vi "Polling Logging Data From PLC.vi"(7 "Polling Data Input":T1, 8 "error in (no error)":errorcluster, 11 "TCP Network Connection in":refnum<k5>) -> (0 "error out":errorcluster, 1 "Data Read":u8[][](array[numeric]), 2 "PLC Data out":T1, 3 "TCP Network Connection out":refnum<k5>, 4 "Elapsed Time(ms)":u32, 5 "Float Data Valid?":bool[](array[boolean]), 6 "Motor2RatingRPM":u16)   [LabVIEW 2018]
uses:
  Ctls/DisplayIndicator.ctl
  Ctls/MotroConfigData.ctl
  Ctls/MotorConfig.ctl
  Ctls/MagType.ctl
  Siemens S7 TCP v3_3 LV 8_5/Siemens S7 TCP v3_3 LV 8_5/S7 TCP API Library/S7 TCP.lvlib
panel:
  out "Motor1RatingRPM":u16
  out "Bool Data Valid":bool
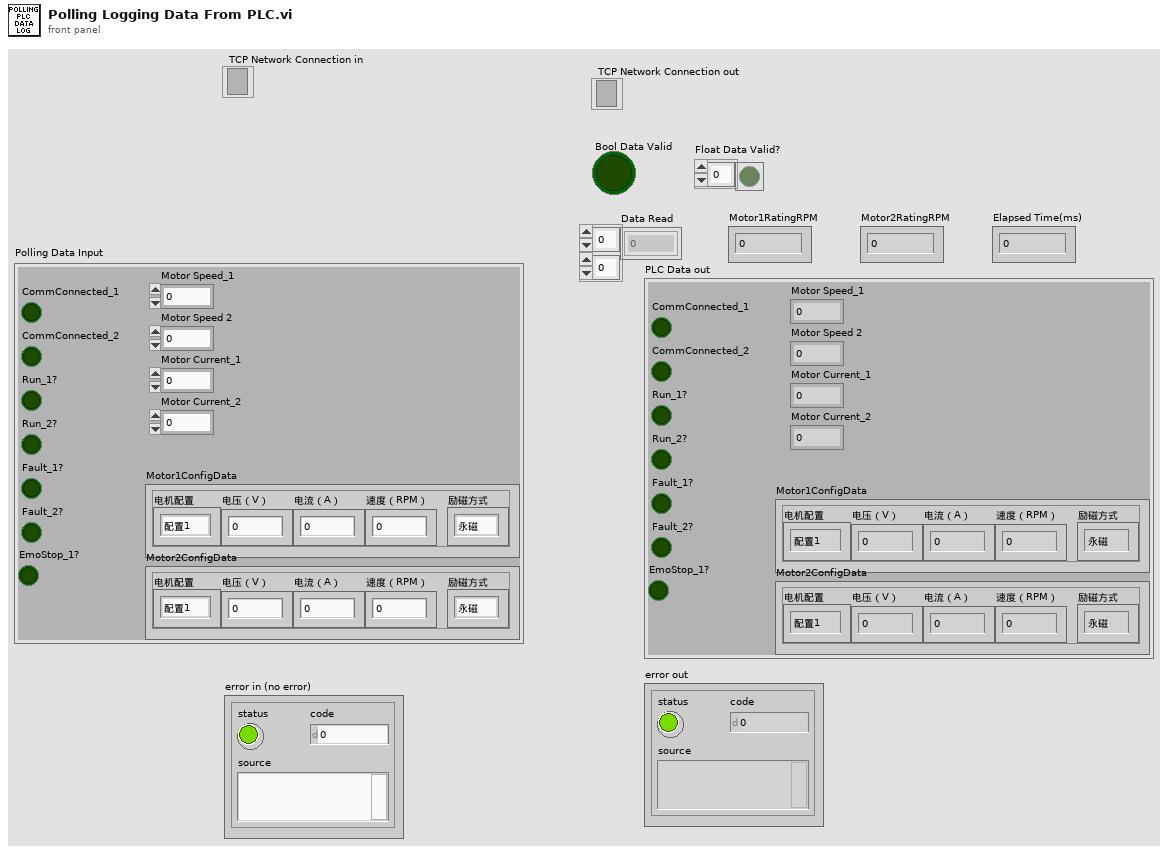
[diagram p1: front panel]
types:
  T1 = typedef "DisplayIndicator.ctl" = cluster{"CommConnected_1":bool, "Run_1?":bool, "Fault_1?":bool, "CommConnected_2":bool, "Run_2?":bool, "Fault_2?":bool, "Motor Speed 2":sgl, "Motor Speed_1":sgl, "Motor Current_1":sgl, "Motor Current_2":sgl, "Motor1ConfigData":T2, "Motor2ConfigData":T2, "EmoStop_1?":bool}
  T2 = typedef "MotroConfigData.ctl" = cluster{"电机配置":T3, "电压（V）":dbl, "电流（A）":dbl, "速度（RPM）":dbl, "励磁方式":T4}
  T3 = typedef "MotorConfig.ctl" = enum16{"配置1", "配置2", "配置3", "配置4"}
  T4 = typedef "MagType.ctl" = enum16{"永磁", "励磁"}
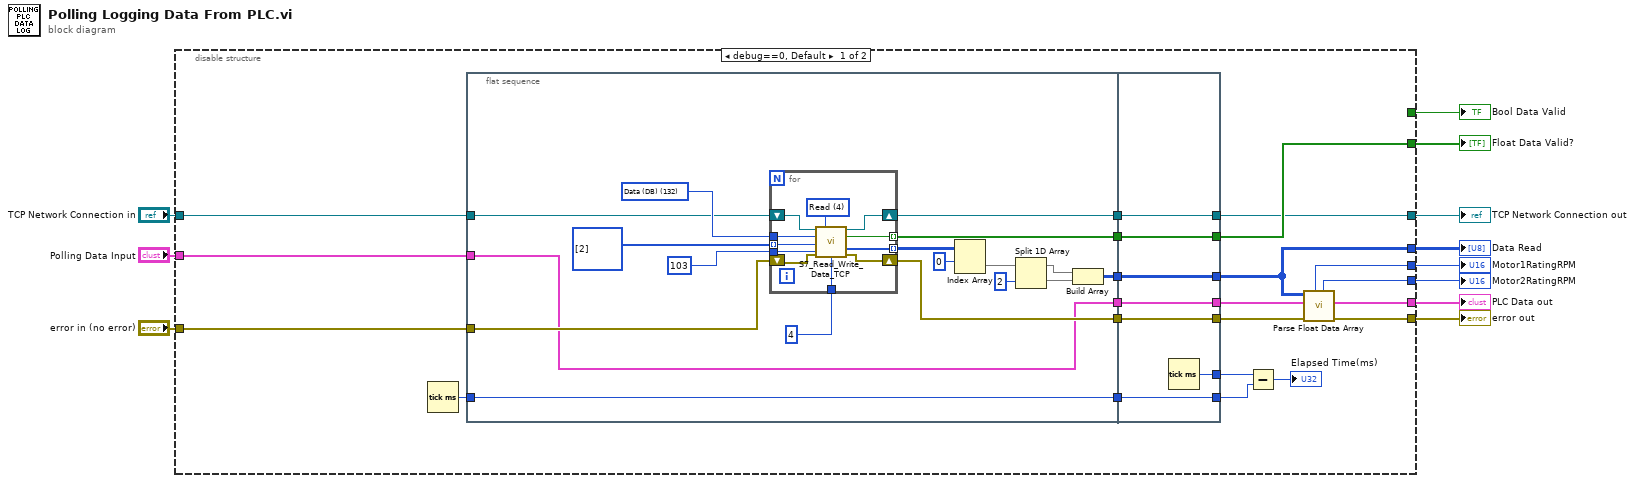
[diagram p0: block diagram]
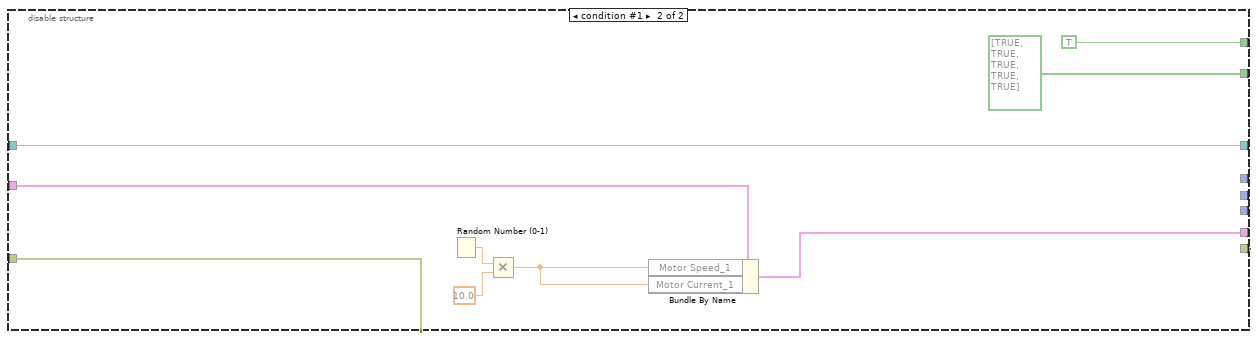
[diagram p2: hidden frame]
diagram:
  n1 = disable-structure shown="debug==0, Default" {
    disable-tunnel: [w33 w75] -> w11
    disable-tunnel: [w32 w71] -> w10
    disable-tunnel: [w24 _] -> w9
    disable-tunnel: [w31 bool[] [TRUE, TRUE, TRUE, TRUE, TRUE]] -> w8
    disable-tunnel: [w30 w78] -> w7
    disable-tunnel: [_ TRUE ("Data Valid")] -> w6
    disable-tunnel: "TCP Network Connection in" -> [w27 w78]
    disable-tunnel: "error in (no error)" -> [w25 w71]
    disable-tunnel: [w29 _] -> w3
    disable-tunnel: [w28 _] -> w2
    disable-tunnel: "Polling Data Input" -> [w23 w70]
    frame condition #0 (active) {
      n2 = Tick Count (ms)() -> (millisecond timer value=w16:u32)
      n3 = flat-sequence {
        tunnel: w27 -> [w45]
        tunnel: w25 -> [w43]
        tunnel: w23 -> [w35]
        tunnel: [w51] -> w21
        tunnel: [w48] -> w20
        tunnel: [w44] -> w19
        tunnel: [w36] -> w18
        tunnel: [w35] -> w17
        tunnel: w16 -> [w34]
        tunnel: [w34] -> w15
        tunnel: [w65] -> w22
        tunnel: [w66] -> w24
        tunnel: [w67] -> w26
        tunnel: [w68] -> w30
        tunnel: [w69] -> w31
        tunnel: w21 -> [w69]
        tunnel: w20 -> [w68]
        tunnel: w19 -> [w67]
        tunnel: w18 -> [w66]
        tunnel: w17 -> [w65]
        tunnel: [w64] -> w14
        tunnel: w15 -> [w63]
        tunnel: [w63] -> w13
        frame #0 {
          w47 = u8 132 items=["I/O (P)"=128, "Input (I)"=129, "Output (Q)"=130, "Bit Memory (M)"=131, "Data (DB)"=132, "Instance Data (DI)"=133, "Local Data (L)"=134, "Predecessor Local Data (VL)"=135] ("Address Areas")
          n4 = for {
            tunnel: w47 -> [w61]
            tunnel: u16 103 ("Data Block #") -> [w58]
            tunnel: u32[] [2] -> [w57] mode=indexing
            tunnel: u16 4 ("Length (bytes)") -> [w56]
            tunnel: [w55] -> w51 mode=indexing
            tunnel: [w54] -> w42 mode=indexing
            shift-right: [w52] -> w44
            shift-left: w43 -> [w53]
            shift-right: [w59] -> w48
            shift-left: w45 -> [w62]
            w60 = u8 4 items=["Read"=4, "Write"=5] ("Read / Write")
            n5 = call "S7_Read_Write_Data_TCP.vi"("TCP Connection Ref"=w62, "Read / Write"=w60, "Address Areas"=w61, "Start Address (bytes)"=w57, "Data Block #"=w58, "error in"=w53, "Length (bytes)"=w56) -> ("TCP Connection Ref Out"=w59:refnum<k5>, "Data Valid"=w55:bool, "Data Read"=w54:u8[], "error out"=w52:errorcluster)  [unwired: 3 in, 2 out]
          }
          n6 = Index Array(array=w42, index (row)=0) -> (element=w40:u8[])  [unwired: 1 in]
          n7 = Split 1D Array(array=w40, index=2) -> (first subarray=w38:u8[], second subarray=w37:u8[])
          n8 = Build Array(w38, w37) -> (w36:u8[][])
        }
        frame #1 {
          n9 = Tick Count (ms)() -> (millisecond timer value=w64:u32)
        }
      }
      n10 = Subtract(x=w14, y=w13) -> (x-y=→"Elapsed Time(ms)":u32)
      n11 = call "Parse Float Data Array.vi"("error in (no error)"=w26, "PLC Data in"=w22, "Data Read"=w24) -> ("error out"=w32:errorcluster, "PLC Data out"=w33:T1, "Motor2RatingRPM"=w28:u16, "Motor1RatingRPM"=w29:u16)  [unwired: 5 in]
    }
    frame condition #1 {
      n12 = Random Number (0-1)() -> (number: 0 to 1=w74:dbl)
      n13 = Multiply(x=w74, y=10.0) -> (x*y=w72:dbl)
      n14 = Bundle By Name(cluster=w70, "Motor Speed_1"=w72, "Motor Current_1"=w72) -> (w75:T1)
    }
  }
  "Bool Data Valid" <- w6
  "Float Data Valid?" <- w8
  "Data Read" <- w9
  "PLC Data out" <- w11
  "error out" <- w10
  "TCP Network Connection out" <- w7
  "Motor1RatingRPM" <- w3
  "Motor2RatingRPM" <- w2
